vi "ADO Connection Transaction.vi"(8 "error in (no error)":errorcluster caption="错误输入（无错误）", 9 "isolation level (chaos)":T1, 10 "operation (begin)":T2, 11 "Database Connection 输入":refnum<class "Database Connection.lvclass"> caption="DNL_LabVIEW Object in") -> (0 "error out":errorcluster caption="错误输出", 1 "ADO isolation level":i32(ring)=-1 items=["adXactUnspecified"=-1, "adXactChaos"=16, "adXactReadUncommitted, adXactBrowse"=256, "adXactCursorStability, adXactReadCommitted"=4096, "adXactRepeatableRead"=65536, "adXactSerializable, adXactIsolated"=1048576], 3 "Database Connection 输出":refnum<class "Database Connection.lvclass"> caption="DNL_LabVIEW Object out")   [LabVIEW 2011, in "Database Connection.lvclass"]
uses:
  Database Connection.lvclass
  <vilib>/addons/database/Auxilliary.llb/DB Tools Transaction.ctl
  <vilib>/addons/database/Auxilliary.llb/DB Tools Isolation Level.ctl
  Database Connection.lvclass/Database Connection.ctl
  <vilib>/addons/database/NI_Database_API.lvlib
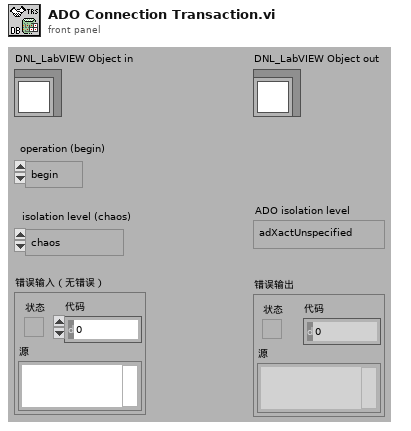
[diagram p1: front panel]
types:
  T1 = typedef "NI_Database_API.lvlib/DB Tools Isolation Level.ctl" = enum16{"chaos", "read uncommitted", "read committed", "repeatable read", "serializable"}
  T2 = typedef "NI_Database_API.lvlib/DB Tools Transaction.ctl" = enum16{"begin", "commit", "rollback"}
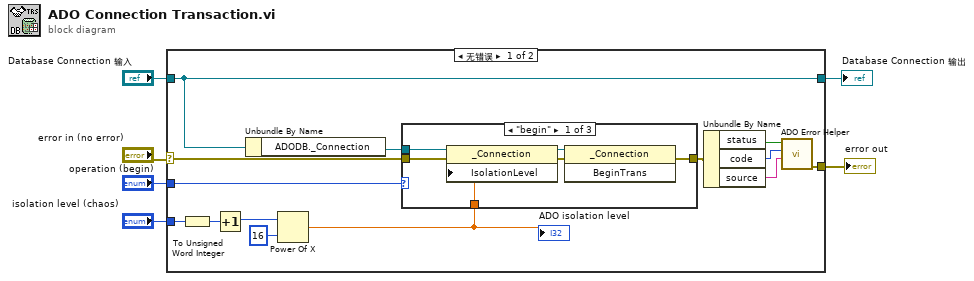
[diagram p0: block diagram]
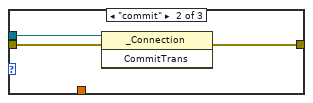
[diagram p2: hidden frame]
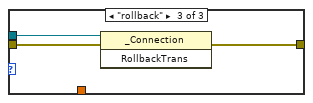
[diagram p3: hidden frame]
diagram:
  n1 = case shown="无错误" "error in (no error)" {
    selector: "error in (no error)" -> [w13 w34]
    tunnel: [w9 w34] -> w5
    tunnel: [w15 w33] -> w3
    tunnel: "Database Connection 输入" -> [w15 w33]
    tunnel: "isolation level (chaos)" -> [w16 _]
    tunnel: "operation (begin)" -> [w7 _]
    frame No Error {
      n2 = To Unsigned Word Integer(number=w16) -> (unsigned 16bit integer=w18:u16)
      n3 = Increment(x=w18) -> (x+1=w19:u16)
      n4 = Unbundle By Name(w15) -> ("ADODB._Connection"=w14:refnum<k7>)
      n5 = Power Of X(1:u16 16 ("x"), 2:w19) -> (0:w8:dbl)
      "ADO isolation level" <- w8
      n6 = case shown="\"begin\"" w7 {
        tunnel: [w26 w29 w32] -> w20
        tunnel: w14 -> [w25 w28 w31]
        tunnel: w8 -> [w22 _ _]
        tunnel: w13 -> [w21 w27 w30]
        frame "begin" {
          n7 = property class="_Connection"(reference=w25, error in=w21, "IsolationLevel"=w22) -> (reference out=w24:refnum<k7>, error out=w23:errorcluster)
          n8 = invoke class="_Connection" method="BeginTrans"(reference=w24, error in=w23) -> (error out=w26:errorcluster)  [unwired: 1 in, 2 out]
        }
        frame "commit" {
          n9 = invoke class="_Connection" method="CommitTrans"(reference=w28, error in=w27) -> (error out=w29:errorcluster)  [unwired: 1 in, 2 out]
        }
        frame "rollback" {
          n10 = invoke class="_Connection" method="RollbackTrans"(reference=w31, error in=w30) -> (error out=w32:errorcluster)  [unwired: 1 in, 2 out]
        }
      }
      n11 = Unbundle By Name(w20) -> ("status"=w12:bool, "code"=w11:i32, "source"=w10:string)
      n12 = call "ADO Error Helper.vi"("source"=w10, "code"=w11, "status"=w12) -> ("error out"=w9:errorcluster)  [unwired: 8 in]
    }
    frame Error {
    }
  }
  "error out" <- w5
  "Database Connection 输出" <- w3
